vi "Proiect_2.vi"() -> ()   [LabVIEW 2024]
uses:
  <vilib>/Instr/_visa.llb/VISA Configure Serial Port (Instr).vi
panel:
  in  "Anul":dbl=2025.0
  in  "Luna":dbl=4.0
  in  "Ziua":dbl=26.0
  out "Datele citite":dbl[](graph)
  in  "Selectare Valoare Citita":u16(ring)=3 items=["Temperatura", "Umiditate", "Valoare MQ3", "Valoare MQ5", "Indice Comfort Termic"]
  in  "Selectarea Numarului de valori citite din istoric":dbl=20.0
  out "Indice Comfort Termic":dbl=77.75473
  in  "?":bool
  in  "Interval de salvare [min]":dbl=0.2
  in  "Interval de masurare [sec]":dbl=3.0
  out "Grafic":waveform(dbl)(graph)={"t0"=timestamp(3832057380.1724057 s since 1904-01-01), "dt"=1.0, "Y"=[102.0]}
  out "Valoarea curenta":dbl=102.0
  in  "Selectare Valoare Grafic":u16(ring)=3 items=["Temperatura", "Umiditate", "Valoare MQ3", "Valoare MQ5", "Indice Comfort Termic"]
  out "Valoare MQ5":dbl=102.0
  out "Valoare MQ3":dbl=252.0
  out "Temperatura":dbl=26.7
  out "Umiditate":dbl=81.0
  out "Citirea din Buffer":string="Humidity: 81.00 Temperature: 26.70 Valoare gaz MQ3: 252.00 Valoare gaz MQ5: 102.00\r\n"
  in  "?":bool
  in  "Port-ul folosit":refnum<visa-resource-name>="COM3"
  # "Pentru citirea corecta a datelor, trebuie introdus\n un interval de masurare de cel putin 3 secunde!\n(Daca se citeste zero la toti parametrii inseamna ca a aparut o citire gresita)"
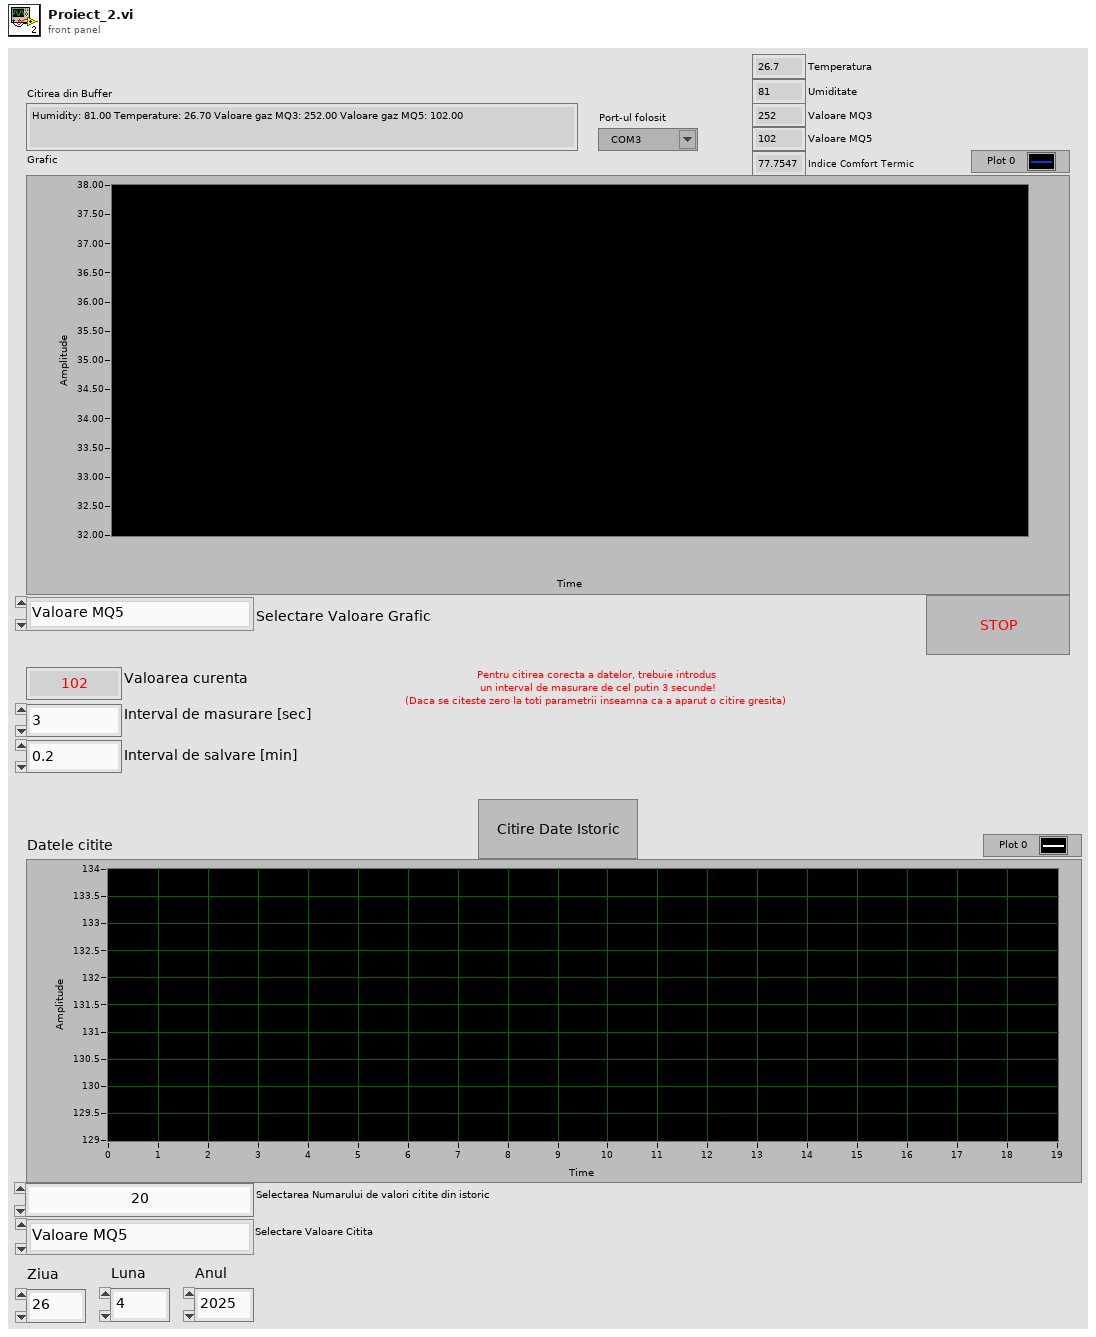
[diagram p1: front panel]
types:
  T1 = enum16{"open", "replace", "create", "open or create", "replace or create", "replace or create with confirmation"}
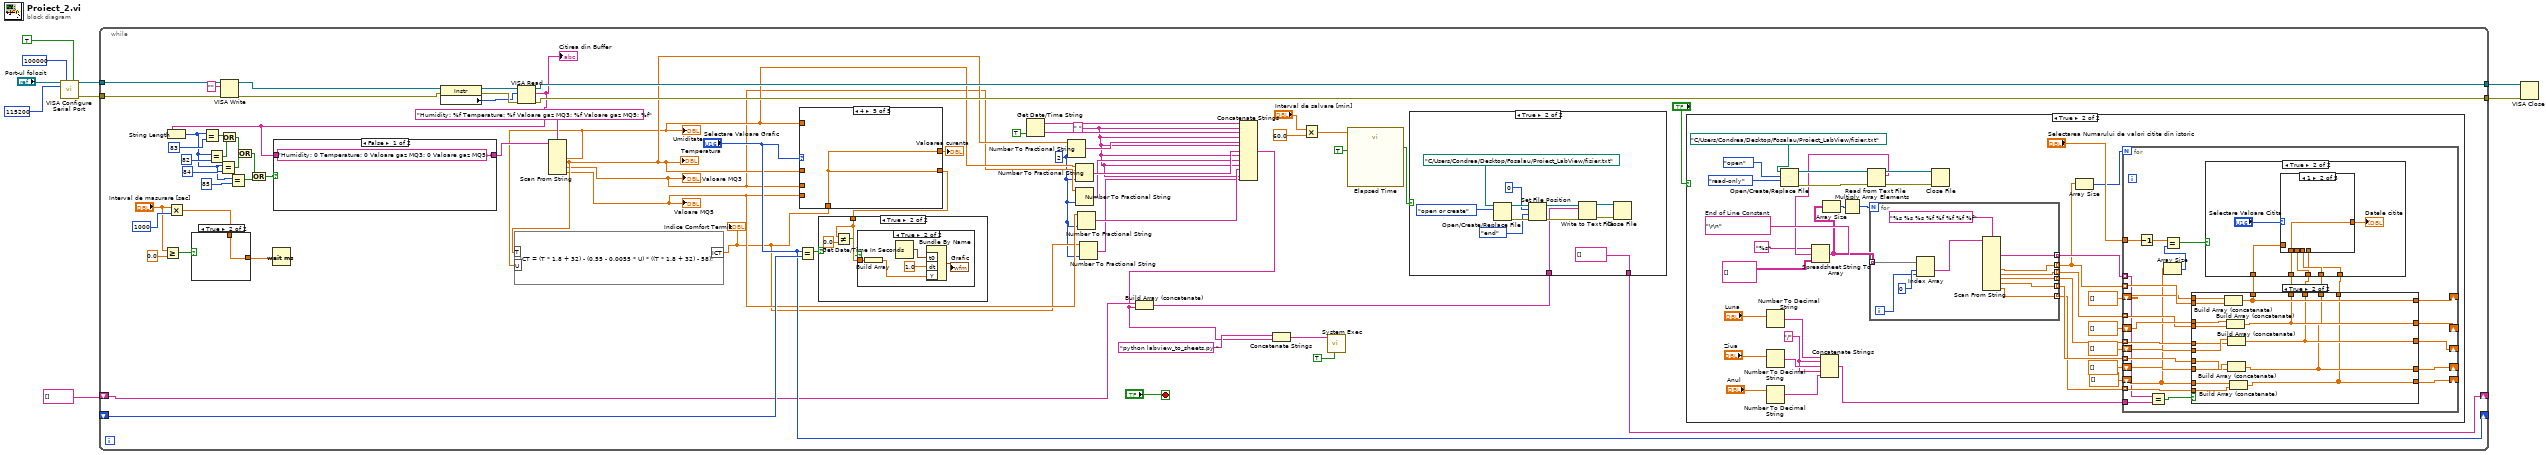
[diagram p0: block diagram]
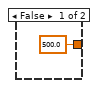
[diagram p10: hidden frame]
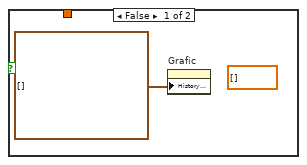
[diagram p12: hidden frame]
diagram:
  n1 = call-poly "VISA Configure Serial Port"("VISA resource name"="Port-ul folosit", "timeout (10sec)"=u32 100000, "Enable Termination\nChar (T)"=TRUE ("Enable Termination\nChar (T)"), "baud rate (9600)"=u32 115200) -> ("VISA resource name out"=w7:refnum<visa-resource-name>, "error out"=w6:errorcluster)  [unwired: 10 in]
  n2 = while {
    tunnel: w7 -> [w74]
    tunnel: w6 -> [w73]
    tunnel: [w67] -> w5
    tunnel: [w66] -> w4
    shift-right: ["Selectare Valoare Grafic"] -> _
    shift-left: _ -> [w62]
    shift-right: [w15] -> _
    shift-left: string[] [] -> [w16]
    stop <- "?" stop-if-true
    w19 = i16 2 ("precision (6)")
    w18 = " " ("string")
    n3 = Greater Or Equal?(x="Interval de masurare [sec]", y=0.0) -> (x >= y?=w41:bool)
    n4 = Multiply(x="Interval de masurare [sec]", y=u32 1000) -> (x*y=w39:dbl)
    n5 = case shown="True" w41 {
      tunnel: [500.0 w194] -> w38
      tunnel: w39 -> [_ w194]
      frame False {
      }
      frame True {
      }
    }
    n6 = VISA Write(VISA resource name=w74, write buffer="", error in (no error)=w73) -> (VISA resource name out=w72:refnum<visa-resource-name>, error out=w71:errorcluster)  [unwired: 1 out]
    n7 = Wait (ms)(milliseconds to wait=w38) -> ()  [unwired: 1 out]
    n8 = property class="Instr"(reference=w72, error in=w71) -> (reference out=w70:refnum<visa-resource-name>, error out=w69:errorcluster, "Serial Settings:Number of Bytes at Serial Port"=w68:u32)
    n9 = VISA Read(VISA resource name=w70, byte count=w68, error in (no error)=w69) -> (VISA resource name out=w67:refnum<visa-resource-name>, read buffer=w51:string, error out=w66:errorcluster)  [unwired: 1 out]
    "Citirea din Buffer" <- w51
    n10 = String Length(string=w51) -> (length=w48:i32)
    n11 = Equal?(x=w48, y=83) -> (x = y?=w57:bool)
    n12 = Equal?(x=w48, y=82) -> (x = y?=w55:bool)
    n13 = Equal?(x=w48, y=84) -> (x = y?=w52:bool)
    n14 = Or(x=w57, y=w55) -> (x .or. y?=w54:bool)
    n15 = Equal?(x=w48, y=85) -> (x = y?=w46:bool)
    n16 = Or(x=w54, y=w52) -> (x .or. y?=w49:bool)
    n17 = Or(x=w49, y=w46) -> (x .or. y?=w45:bool)
    n18 = case shown="False" w45 {
      tunnel: w51 -> [_ w196]
      tunnel: ["Humidity: 0 Temperature: 0 Valoare gaz MQ3: 0 Valoare gaz MQ5: 0" ("read buffer") w196] -> w50
      frame False {
      }
      frame True {
      }
    }
    n19 = Scan From String(format string="Humidity: %f Temperature: %f Valoare gaz MQ3: %f Valoare gaz MQ5: %f", input string=w50) -> (output 1=w34:dbl, output 2=w36:dbl, output 3=w31:dbl, output 4=w30:dbl)  [unwired: 6 in, 3 out]
    "Umiditate" <- w34
    "Temperatura" <- w36
    "Valoare MQ3" <- w31
    "Valoare MQ5" <- w30
    n20 = formula code="ICT = (T * 1.8 + 32) - (0.55 - 0.0055 * U) * ((T * 1.8 + 32) - 58);"("T"=w36, "U"=w34) -> ("ICT"=w20:dbl)
    "Indice Comfort Termic" <- w20
    n21 = Equal?(x="Selectare Valoare Grafic", y=w62) -> (x = y?=w60:bool)
    n22 = case shown="4" "Selectare Valoare Grafic" {
      tunnel: [w206 w207 w208 w209 w210] -> w59
      tunnel: w36 -> [w206 _ _ _ _]
      tunnel: w34 -> [_ w207 _ _ _]
      tunnel: w31 -> [_ _ w208 _ _]
      tunnel: w30 -> [_ _ _ w209 _]
      tunnel: [w206 w207 w208 w209 w210] -> w63
      tunnel: w20 -> [_ _ _ _ w210]
      frame 0, Default {
      }
      frame 1 {
      }
      frame 2 {
      }
      frame 3 {
      }
      frame 4 {
      }
    }
    "Valoarea curenta" <- w63
    n23 = case shown="True" w60 {
      tunnel: w59 -> [_ w200]
      frame False {
        (unwired) dbl[] []
        n24 = property on="Grafic" class="WFChart (strict)"("History Data"=waveform(dbl)[] []) -> ()  [unwired: 2 in, 2 out]
      }
      frame True {
        n25 = Not Equal?(x=w200, y=0.0) -> (x != y?=w198:bool)
        n26 = case shown="True" w198 {
          tunnel: w200 -> [_ w205]
          frame False {
          }
          frame True {
            n27 = Build Array(w205) -> (w201:dbl[])
            n28 = Get Date/Time In Seconds() -> (seconds since 1Jan1904=w203:timestamp)
            n29 = Bundle By Name("t0"=w203, "dt"=1.0, "Y"=w201) -> (→"Grafic":waveform(dbl))  [unwired: 1 in]
          }
        }
      }
    }
    n30 = Get Date/Time String(want seconds? (F)=TRUE) -> (date string=w44:string, time string=w43:string)  [unwired: 2 in]
    n31 = Number To Fractional String(number=w36, precision (6)=w19) -> (F-format string=w35:string)  [unwired: 2 in]
    n32 = Number To Fractional String(number=w31, precision (6)=w19) -> (F-format string=w32:string)  [unwired: 2 in]
    n33 = Number To Fractional String(number=w34, precision (6)=w19) -> (F-format string=w33:string)  [unwired: 2 in]
    n34 = Number To Fractional String(number=w30, precision (6)=w19) -> (F-format string=w29:string)  [unwired: 2 in]
    n35 = Number To Fractional String(number=w20, precision (6)=w19) -> (F-format string=w17:string)  [unwired: 2 in]
    n36 = Concatenate Strings(w44, w18, w43, w18, w35, w18, w33, w18, w32, w18, w29, w18, w17) -> (w12:string)
    n37 = Build Array (concatenate)(w16, w12) -> (w14:string[])
    n38 = Concatenate Strings("python labview_to_sheets.py " ("string"), w12) -> (w11:string)
    n39 = Multiply(x="Interval de salvare [min]", y=60.0) -> (x*y=w24:dbl)
    n40 = call <vilib>:"System Exec.vi"("run minimized? (F)"=TRUE, "command line"=w11) -> ()  [unwired: 6 in, 4 out]
    n41 = call "Elapsed Time"("Time Target (s)"=w24, "Auto Reset"=TRUE) -> ("Time has Elapsed"=w22:bool)  [unwired: 10 in, 7 out]
    n42 = case shown="True" w22 {
      tunnel: w14 -> [w180 w182]
      tunnel: [w180 string[] []] -> w15
      frame False {
      }
      frame True {
        n43 = Open/Create/Replace File(file path (use dialog)=path "C:/Users/Condrea/Desktop/Fosalau/Proiect_LabView/fisier.txt", operation (0:open)=T1."open or create") -> (refnum out=w187:refnum<file>, error out=w188:errorcluster)  [unwired: 4 in, 1 out]
        n44 = Set File Position(offset (in bytes) (0)=i64 0, refnum=w187, from (0:start)=enum16{"start", "end", "current"}."end", error in=w188) -> (refnum out=w183:refnum<file>, error out=w184:errorcluster)
        n45 = Write to Text File(file (use dialog)=w183, text=w182, error in=w184) -> (refnum out=w192:refnum<file>, error out=w191:errorcluster)  [unwired: 1 in, 1 out]
        n46 = Close File(refnum=w192, error in=w191) -> ()  [unwired: 2 out]
      }
    }
    n47 = case shown="True" "?" {
      frame False {
      }
      frame True {
        w80 = "/" ("string")
        w102 = "\r\n"  # End of Line Constant
        n48 = Number To Decimal String(number="Luna") -> (decimal integer string=w82:string)  [unwired: 1 in]
        n49 = Number To Decimal String(number="Ziua") -> (decimal integer string=w81:string)  [unwired: 1 in]
        n50 = Number To Decimal String(number="Anul") -> (decimal integer string=w79:string)  [unwired: 1 in]
        n51 = Open/Create/Replace File(file path (use dialog)=path "C:/Users/Condrea/Desktop/Fosalau/Proiect_LabView/fisier.txt" ("file (use dialog)"), operation (0:open)=T1."open", access (0:read/write)=enum16{"read/write", "read-only", "write-only"}."read-only") -> (refnum out=w106:refnum<file>, error out=w107:errorcluster)  [unwired: 3 in, 1 out]
        n52 = Concatenate Strings(w82, w80, w81, w80, w79) -> (w78:string)
        n53 = Read from Text File(file (use dialog)=w106, error in=w107) -> (refnum out=w105:refnum<file>, text=w101:string, error out=w104:errorcluster)  [unwired: 2 in, 1 out]
        n54 = Spreadsheet String To Array(delimiter (Tab)=w102, format string="%s", spreadsheet string=w101, array type (2D Dbl)=string[][] []) -> (array=w97:string[][])
        n55 = Array Size(array=w97) -> (size(s)=w98:i32[])
        n56 = Multiply Array Elements(1:w98) -> (0:w96:i32)
        n57 = for {
          N: w96 -> [_]
          tunnel: w97 -> [w179] mode=indexing
          tunnel: [w176] -> w90 mode=indexing
          tunnel: [w173] -> w76 mode=indexing
          tunnel: [w172] -> w93 mode=indexing
          tunnel: [w171] -> w91 mode=indexing
          tunnel: [w170] -> w89 mode=indexing
          tunnel: [w169] -> w77 mode=indexing
          i -> [w174]
          n58 = Index Array "Index Array"(array=w179, index #1=0 ("index"), index #2=w174) -> (element #1=w178:string)  [unwired: 1 out]
          n59 = Scan From String "Scan From String"(format string="%s %s %s %f %f %f %f %f", input string=w178) -> (output 1=w169:string, output 4=w173:dbl, output 5=w172:dbl, output 6=w171:dbl, output 7=w176:dbl, output 8=w170:dbl)  [unwired: 12 in, 3 out]
        }
        n60 = Close File(refnum=w105, error in=w104) -> ()  [unwired: 2 out]
        n61 = Array Size(array=w76) -> (size(s)=w75:i32)
        n62 = for {
          N: w75 -> [_]
          tunnel: w76 -> [w132] mode=indexing
          tunnel: "Selectarea Numarului de valori citite din istoric" -> [w136]
          shift-right: [w134] -> _
          shift-left: dbl[] [] -> [w131]
          shift-right: [w123] -> _
          shift-left: dbl[] [] -> [w130]
          tunnel: w93 -> [w129] mode=indexing
          tunnel: w91 -> [w127] mode=indexing
          tunnel: w90 -> [w125] mode=indexing
          tunnel: w89 -> [w124] mode=indexing
          shift-right: [w122] -> _
          shift-left: dbl[] [] -> [w128]
          shift-right: [w121] -> _
          shift-left: dbl[] [] -> [w126]
          shift-right: [w120] -> _
          shift-left: dbl[] [] -> [w117]
          tunnel: w78 -> [w119]
          tunnel: w77 -> [w110] mode=indexing
          n63 = Decrement(x=w136) -> (x-1=w133:dbl)
          n64 = Equal?(x=w110, y=w119) -> (x = y?=w118:bool)
          n65 = Array Size(array=w117) -> (size(s)=w116:i32)
          n66 = Equal?(x=w133, y=w116) -> (x = y?=w135:bool)
          n67 = case shown="True" w118 {
            tunnel: [w141 w146] -> w134
            tunnel: w132 -> [_ w156]
            tunnel: w131 -> [w141 w155]
            tunnel: w130 -> [w140 w154]
            tunnel: w129 -> [_ w153]
            tunnel: w128 -> [w139 w152]
            tunnel: w127 -> [_ w151]
            tunnel: w126 -> [w138 w150]
            tunnel: w125 -> [_ w149]
            tunnel: w117 -> [w137 w148]
            tunnel: w124 -> [_ w147]
            tunnel: [w140 w145] -> w123
            tunnel: [w139 w144] -> w122
            tunnel: [w138 w143] -> w121
            tunnel: [w137 w142] -> w120
            tunnel: [w141 w146] -> w115
            tunnel: [w140 w145] -> w114
            tunnel: [w139 w144] -> w113
            tunnel: [w138 w143] -> w112
            tunnel: [w137 w142] -> w111
            frame False {
            }
            frame True {
              n68 = Build Array (concatenate)(w155, w156) -> (w146:dbl[])
              n69 = Build Array (concatenate)(w154, w153) -> (w145:dbl[])
              n70 = Build Array (concatenate)(w152, w151) -> (w144:dbl[])
              n71 = Build Array (concatenate)(w150, w149) -> (w143:dbl[])
              n72 = Build Array (concatenate)(w148, w147) -> (w142:dbl[])
            }
          }
          n73 = case shown="True" w135 {
            tunnel: w115 -> [_ w161]
            tunnel: w114 -> [_ w160]
            tunnel: w113 -> [_ w159]
            tunnel: w112 -> [_ w158]
            tunnel: w111 -> [_ w157]
            frame False {
            }
            frame True {
              n74 = case shown="1" "Selectare Valoare Citita" {
                tunnel: [w164 w165 w166 w167 w168] -> w162
                tunnel: w161 -> [w164 _ _ _ _]
                tunnel: w160 -> [_ w165 _ _ _]
                tunnel: w159 -> [_ _ w166 _ _]
                tunnel: w158 -> [_ _ _ w167 _]
                tunnel: w157 -> [_ _ _ _ w168]
                frame 0, Default {
                }
                frame 1 {
                }
                frame 2 {
                }
                frame 3 {
                }
                frame 4 {
                }
              }
              "Datele citite" <- w162
            }
          }
        }
      }
    }
  }
  n75 = VISA Close(VISA resource name=w5, error in (no error)=w4) -> ()  [unwired: 1 out]
